vi "Read Tag.vi"(8 "error in (no error)":errorcluster, 11 "Enum":T1) -> (0 "error out":errorcluster, 3 "value":string)   [LabVIEW 2025, in "Full User Interface.lvlib"]
uses:
  Full User Interface.lvlib
  Key.ctl
  <vilib>/Utility/config.llb/Read Key (String).vi
  <vilib>/Utility/config.llb/NI_LVConfig.lvlib
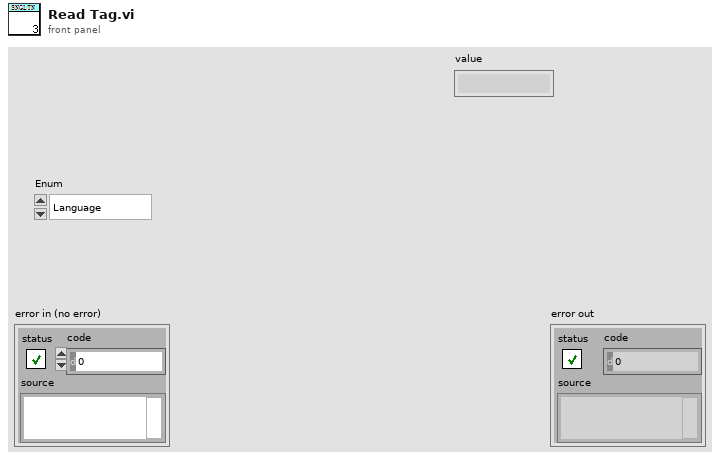
[diagram p1: front panel]
types:
  T1 = typedef "Full User Interface.lvlib/Key.ctl" = enum16{"Language", "Model"}
  T2 = typedef "NI_LVConfig.lvlib/Config Data RefNum.ctl" = refnum<k1>
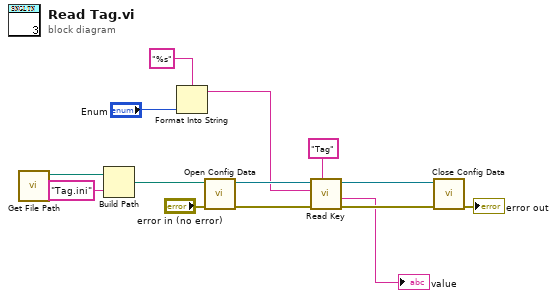
[diagram p0: block diagram]
diagram:
  n1 = call "Get File Path.vi"() -> ("Application Directory"=w14:path)  [unwired: 11 in]
  n2 = Build Path(base path=w14, name or relative path="Tag.ini") -> (appended path=w12:path)
  n3 = Format Into String(format string="%s", "Enum") -> (resulting string=w2:string)  [unwired: 2 in, 1 out]
  n4 = call <vilib>:"Open Config Data.vi"("error in (no error)"="error in (no error)", "configuration file path"=w12) -> ("error out"=w10:errorcluster, "refnum"=w11:T2)  [unwired: 7 in, 1 out]
  n5 = call-poly <vilib>:"Read Key.vi"("section"="Tag", "error in (no error)"=w10, "key"=w2, "refnum"=w11) -> ("error out"=w7:errorcluster, "value"=→"value":string, "refnum out"=w8:T2)  [unwired: 4 in, 1 out]
  n6 = call <vilib>:"Close Config Data.vi"("error in (no error)"=w7, "refnum"=w8) -> ("error out"=→"error out":errorcluster)  [unwired: 8 in, 1 out]
